vi "PRIME Detector Process File.vi"(6 "Image Type":string, 8 "error in (no error)":errorcluster, 9 "Frame":i32, 10 "Camera":i32, 11 "Filename":string) -> (0 "error out":errorcluster, 2 "Keep?":bool, 3 "Image Data":T1)   [LabVIEW 2024]
uses:
  Detector Image typedef cluster.ctl
  Detector Class.lvclass
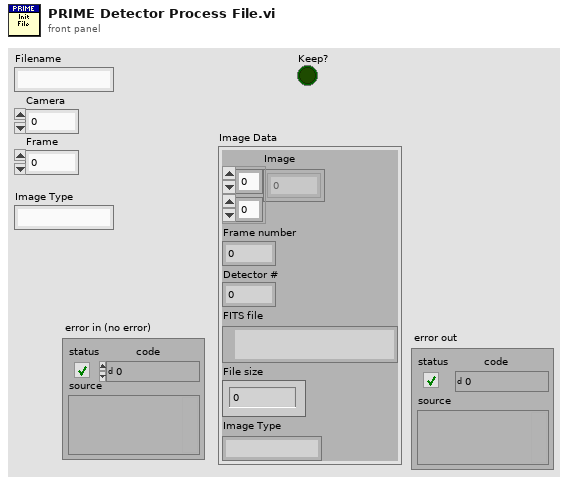
[diagram p1: front panel]
types:
  T1 = typedef "Detector Class.lvclass/Detector Image typedef cluster.ctl" = cluster{"Image":sgl[][], "Frame number":i32, "Detector #":u16, "FITS file":path, "File size":i64, "Image Type":string}
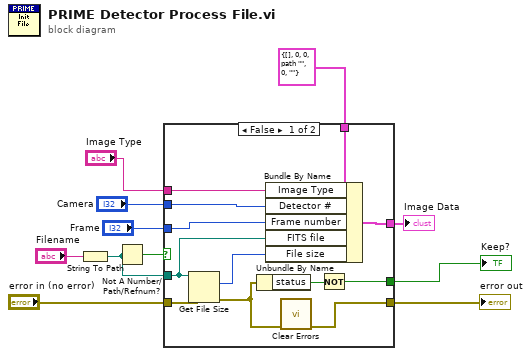
[diagram p0: block diagram]
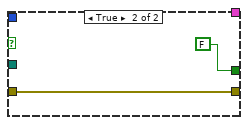
[diagram p2: hidden frame]
diagram:
  n1 = String To Path(string="Filename") -> (path=w11:path)
  n2 = Not A Number/Path/Refnum?(number/path/refnum=w11) -> (NaN/Path/Refnum?=w10:bool)
  n3 = case shown="False" w10 {
    tunnel: T1 {"Image"=[], "Frame number"=0, "Detector #"=0, "FITS file"=path "", "File size"=0, "Image Type"=""} ("Image Data") -> [w23 _]
    tunnel: "Frame" -> [w22 _]
    tunnel: "Camera" -> [w21 _]
    tunnel: [w20 _] -> w2
    tunnel: w11 -> [w13 _]
    tunnel: [w17 FALSE] -> w3
    tunnel: "error in (no error)" -> [w16 w24]
    tunnel: [w15 w24] -> w4
    tunnel: "Image Type" -> [w12 _]
    frame False {
      n4 = Get File Size(file=w13, error in=w16) -> (size (in bytes)=w14:i64, 0:w19:errorcluster)  [unwired: 1 out]
      n5 = Unbundle By Name(w19) -> ("status"=w18:bool)
      n6 = Bundle By Name(cluster=w23, "Image Type"=w12, "Detector #"=w21, "Frame number"=w22, "FITS file"=w13, "File size"=w14) -> (w20:T1)
      n7 = call <vilib>:"Clear Errors.vi"("error in (no error)"=w19) -> ("error out"=w15:errorcluster)  [unwired: 5 in, 1 out]
      n8 = Not(x=w18) -> (.not. x?=w17:bool)
    }
    frame True {
    }
  }
  "error out" <- w4
  "Keep?" <- w3
  "Image Data" <- w2
